vi "Get_Data.vi"(0 "Communication in":refnum<class "Communication.lvclass">, 11 "error in (no error)":errorcluster) -> (4 "Communication out":refnum<class "Communication.lvclass">, 6 "DATA":T1, 15 "error out":errorcluster)   [LabVIEW 2020, in "Data Communication.lvlib" / "Communication.lvclass"]
uses:
  Communication.lvclass
  Typedefs/Data Cluster.ctl
  Communication.lvclass/Communication.ctl
  Data Communication.lvlib
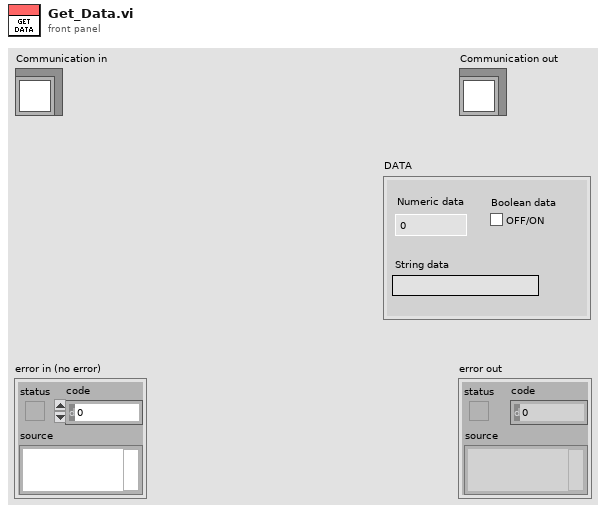
[diagram p1: front panel]
types:
  T1 = typedef "Data Communication.lvlib/Data Cluster.ctl" = cluster{"Numeric data":dbl, "String data":string, "Boolean data":bool}
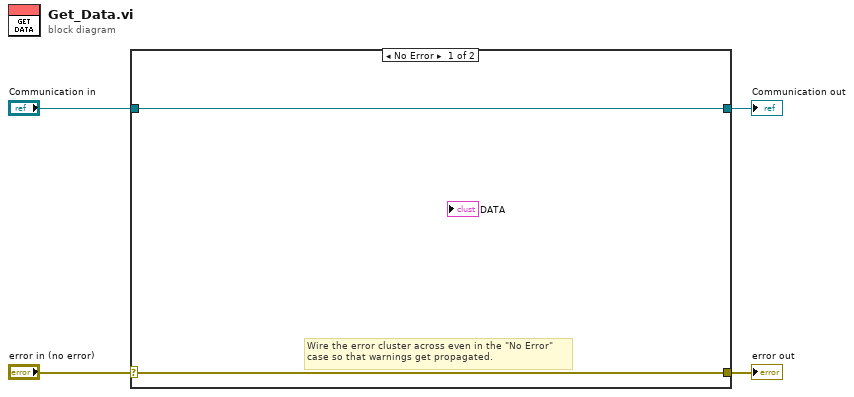
[diagram p0: block diagram]
diagram:
  n1 = case shown="No Error" "error in (no error)" {
    selector: "error in (no error)" -> [w5 w8]
    tunnel: [w5 w8] -> w3
    tunnel: [w6 w7] -> w1
    tunnel: "Communication in" -> [w6 w7]
    frame No Error {
      # "Wire the error cluster across even in the \"No Error\"\ncase so that warnings get propagated."
    }
    frame Error {
    }
  }
  "error out" <- w3
  "Communication out" <- w1
